vi "Configure Signaling RF UL Bandwidth.vi"(8 "error in (no error)":errorcluster, 9 "Bandwidth (5 MHz)":i32(ring) items=["5 MHz", "10 MHz", "15 MHz", "20 MHz", "25 MHz", "30 MHz", "40 MHz", "50 MHz", "60 MHz", "80 MHz", "90 MHz", "100 MHz"], 10 "Cell Name (\"Cell Name\")":string="Cell Name", 11 "VISA resource name":refnum<visa-resource-name>) -> (0 "error out":errorcluster, 3 "VISA resource name out":refnum<visa-resource-name>)   [LabVIEW 2020, in "Rohde&Schwarz CMWXP NR FR1 Measurement.lvlib"]
doc: "Selects the channel bandwidth for the uplink.\n\nAttribute:\nRSCMWXPNRFR1M_ATTR_SIGNALING_RF_UL_BANDWIDTH\n\nRemote-control command:\n[CONFigure:]SIGNaling:NRADio:CELL:RFSettings:UL:BWIDth"
uses:
  <instrlib>/Rohde&Schwarz CMWXP NR FR1 Measurement/Rohde&Schwarz CMWXP NR FR1 Measurement.lvlib
  <instrlib>/Rohde&Schwarz CMWXP NR FR1 Measurement/Private/rsidr_core.llb/rsidr_core.lvlib
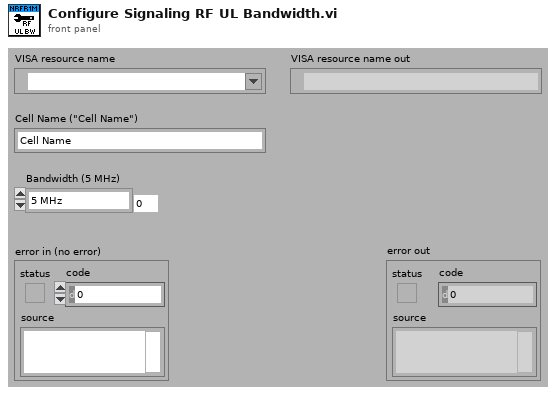
[diagram p1: front panel]
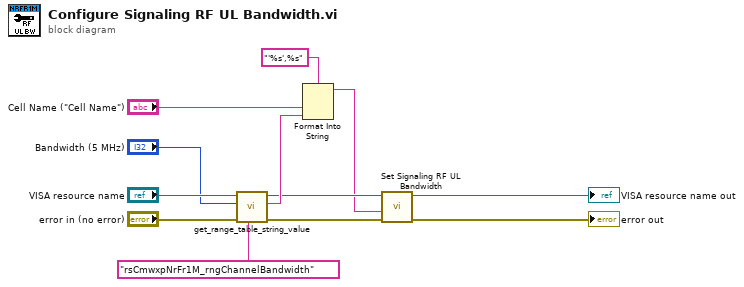
[diagram p0: block diagram]
diagram:
  n1 = call <instrlib>:"get_range_table_string_value.vi"("Range Table ID in"="rsCmwxpNrFr1M_rngChannelBandwidth", "error in"="error in (no error)", "I32 input"="Bandwidth (5 MHz)", "VISA resource name"="VISA resource name") -> ("error out"=w3:errorcluster, "String Value out"=w8:string, "VISA resource name out"=w2:refnum<visa-resource-name>)  [unwired: 5 in]
  n2 = Format Into String(format string="'%s',%s", "Cell Name (\"Cell Name\")", w8) -> (resulting string=w1:string)  [unwired: 2 in, 1 out]
  n3 = call "Set Signaling RF UL Bandwidth"("error in (no error)"=w3, "Signaling RF UL Bandwidth ()"=w1, "instrument handle"=w2) -> ("error out"=→"error out":errorcluster, "instrument handle out"=→"VISA resource name out":refnum<visa-resource-name>)  [unwired: 7 in]
